vi "Encoder to mechanism position.vi"(8 "error in (no error)":errorcluster, 10 "motor position":string, 11 "Motor in":refnum<class "Motor.lvclass">) -> (0 "error out":errorcluster, 2 "mechanism position":string, 3 "Motor out":refnum<class "Motor.lvclass">)   [LabVIEW 2018, in "Motor.lvclass"]
uses:
  Motor.lvclass
  Motor.lvclass/Motor.ctl
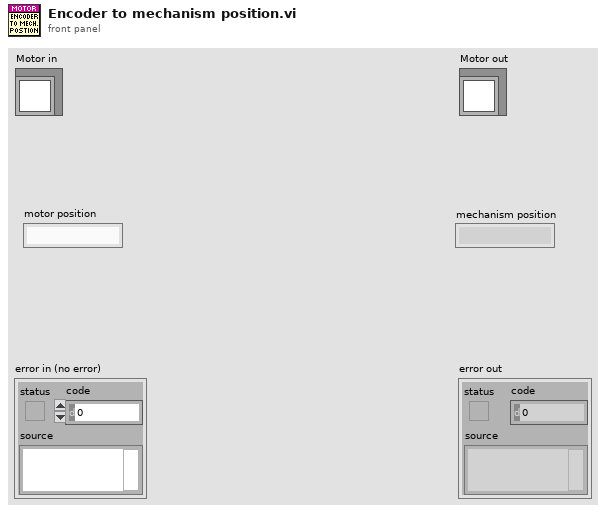
[diagram p1: front panel]
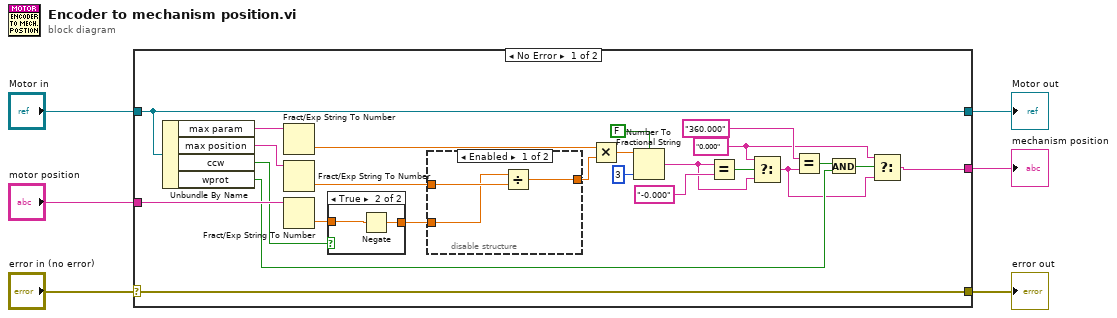
[diagram p0: block diagram]
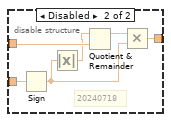
[diagram p2: hidden frame]
diagram:
  n1 = case shown="No Error" "error in (no error)" {
    selector: "error in (no error)" -> [w30 w43]
    tunnel: [w30 w43] -> w5
    tunnel: [w15 w44] -> w3
    tunnel: "Motor in" -> [w15 w44]
    tunnel: "motor position" -> [w24 _]
    tunnel: [w7 _] -> w1
    frame No Error {
      w8 = "0.000"
      n2 = Unbundle By Name(w15) -> ("max param"=w29:string, "max position"=w28:string, "ccw"=w22:bool, "wprot"=w11:bool)
      n3 = Fract/Exp String To Number(string=w29) -> (number=w27:dbl)  [unwired: 3 in, 1 out]
      n4 = Fract/Exp String To Number(string=w28) -> (number=w21:dbl)  [unwired: 3 in, 1 out]
      n5 = Fract/Exp String To Number(string=w24) -> (number=w23:dbl)  [unwired: 3 in, 1 out]
      n6 = case shown="True" w22 {
        tunnel: [w40 w42] -> w14
        tunnel: w23 -> [w40 w41]
        frame False {
        }
        frame True {
          n7 = Negate(x=w41) -> (-x=w42:dbl)
        }
      }
      n8 = disable-structure shown="Enabled" {
        disable-tunnel: w21 -> [w33 w39]
        disable-tunnel: [w32 w36] -> w20
        disable-tunnel: w14 -> [w31 w38]
        frame Enabled {
          n9 = Divide(x=w31, y=w33) -> (x/y=w32:dbl)
        }
        frame Disabled {
          # "20240718"
          n10 = Sign(1:w38) -> (0:w34:dbl)
          n11 = Absolute Value(x=w34) -> (abs(x)=w37:dbl)
          n12 = Quotient & Remainder(x=w37, y=w39) -> (x-y*floor(x/y)=w35:dbl)  [unwired: 1 out]
          n13 = Multiply(x=w35, y=w34) -> (x*y=w36:dbl)
        }
      }
      n14 = Multiply(x=w27, y=w20) -> (x*y=w26:dbl)
      n15 = Number To Fractional String(use system decimal point (T)=FALSE, number=w26, precision (6)=i16 3) -> (F-format string=w16:string)  [unwired: 1 in]
      n16 = Equal?(x=w16, y="-0.000") -> (x = y?=w18:bool)
      n17 = Select(t=w8, s=w18, f=w16) -> (s? t:f=w9:string)
      n18 = Equal?(x="360.000", y=w9) -> (x = y?=w12:bool)
      n19 = And(x=w12, y=w11) -> (x .and. y?=w10:bool)
      n20 = Select(t=w8, s=w10, f=w9) -> (s? t:f=w7:string)
    }
    frame Error {
    }
  }
  "error out" <- w5
  "Motor out" <- w3
  "mechanism position" <- w1
